vi "client.vi"() -> ()   [LabVIEW 2018]
panel:
  in  "header size":i8
  in  "Cluster":cluster{"type":string, "content":string}={"type"="hello", "content"="hello again"}
  out "data out":string
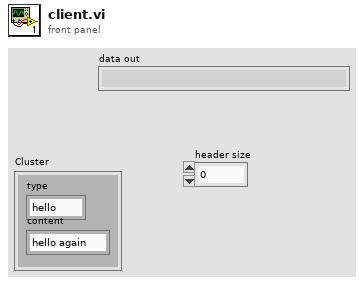
[diagram p1: front panel]
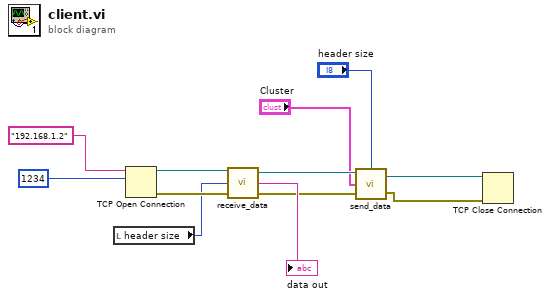
[diagram p0: block diagram]
diagram:
  n1 = local read "header size"() -> (w1:i8)
  n2 = TCP Open Connection(address="192.168.1.2", remote port or service name=u16 1234) -> (connection ID=w10:refnum<k5>, error out=w9:errorcluster)  [unwired: 3 in]
  n3 = call "receive_data.vi"("error in"=w9, "header size"=w1, "connection ID"=w10) -> ("error out"=w5:errorcluster, "data out"=→"data out":string, "connection ID out"=w7:refnum<k5>)
  n4 = call "send_data.vi"("header size"="header size", "error in"=w5, "Cluster"="Cluster", "connection ID"=w7) -> ("error out"=w4:errorcluster, "connection ID out"=w6:refnum<k5>)
  n5 = TCP Close Connection(connection ID=w6, error in (no error)=w4) -> ()  [unwired: 1 in, 2 out]
